vi "Repeat_pulse.vi"(9 "in":i16, 10 "reset":bool, 11 "limit":u16) -> (2 "out":i16, 3 "pulse":bool)   [LabVIEW 2017]
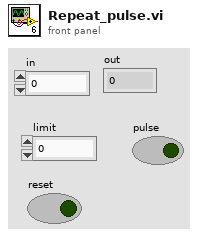
[diagram p1: front panel]
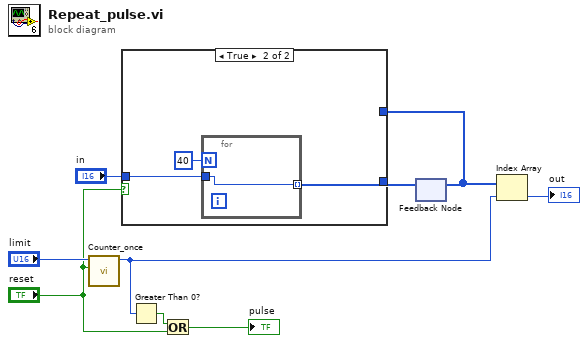
[diagram p0: block diagram]
diagram:
  n1 = call "Counter_once.vi"("reset"="reset", "limit"="limit") -> ("count"=w2:u16)  [unwired: 9 in]
  n2 = Greater Than 0?(x=w2) -> (x > 0?=w8:bool)
  n3 = Or(x=w8, y="reset") -> (x .or. y?=→"pulse":bool)
  n4 = feedback #1() -> (w3:i16[])  [unwired: 1 in]
  n5 = case shown="True" "reset" {
    tunnel: [w10 w12] -> w5
    tunnel: w3 -> [w10 _]
    tunnel: "in" -> [_ w11]
    frame False {
    }
    frame True {
      n6 = for {
        N: 40 -> [_]
        tunnel: [w14] -> w12 mode=indexing
        tunnel: w11 -> [w14]
      }
    }
  }
  n7 = feedback-in #1(w5) -> ()
  n8 = Index Array(array=w3, index=w2) -> (element=→"out":i16)
